vi "Actor Core.vi"(8 "error in":errorcluster, 11 "RandomDataChart in":refnum<class "AutoRegPanel.lvclass">) -> (0 "error out":errorcluster, 3 "Actor out":refnum<class "Actor.lvclass">)   [LabVIEW 2015, in "TestActors.lvlib" / "AutoRegPanel.lvclass"]
doc: "(<B>Filename</B>: Actor Framework.lvlib:Actor.lvclass:Actor Core.vi)\n\nReceives messages to the actor, reacts to them, and initiates any error handling that may shut the actor down.\n\nDescendant classes may override this VI to append parallel tasks for the actor to complete while it handles messages. Overrides use the Call Parent Method node."
uses:
  AutoRegPanel.lvclass
  <vilib>/ActorFramework/Actor/Actor.lvclass
  <vilib>/ActorFramework/Actor/Actor.lvclass/Actor.ctl
  <vilib>/ActorFramework/Message Enqueuer/Message Enqueuer.lvclass/Message Enqueuer.ctl
  <vilib>/ActorFramework/Message Enqueuer/Init from Existing Queue.vi
  IViewable/IViewable/IViewable.lvclass
  <vilib>/ActorFramework/Message Enqueuer/Message Enqueuer.lvclass
  AutoRegistration/AutoRegistration/AutoRegistration.lvclass
  AutoRegistration/ActorAutoRegistration Messages/BooleanValueMsg/BooleanValueMsg.lvclass
panel:
  in  "Whitaker":bool caption="Latch When Released"
  in  "Walton":bool caption="Latch Until Released"
  in  "Launch Dialog":bool
  in  "Guthrie":bool caption="Switch Until Released"
  in  "Harrelson":bool caption="Switch When Released"
  in  "Gump":bool caption="Latch When Pressed"
  in  "Wilson":bool caption="Switch When Pressed"
  # "An actor implementing\ngeneral auto-reg in core"
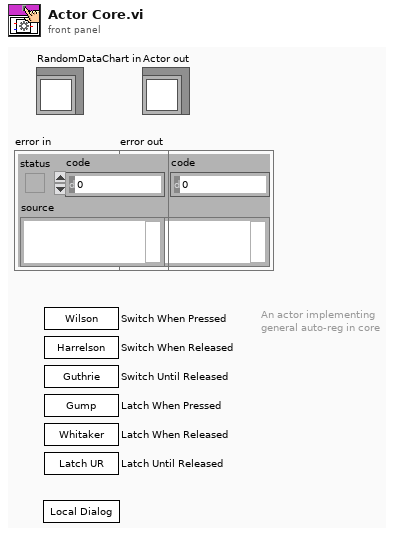
[diagram p1: front panel]
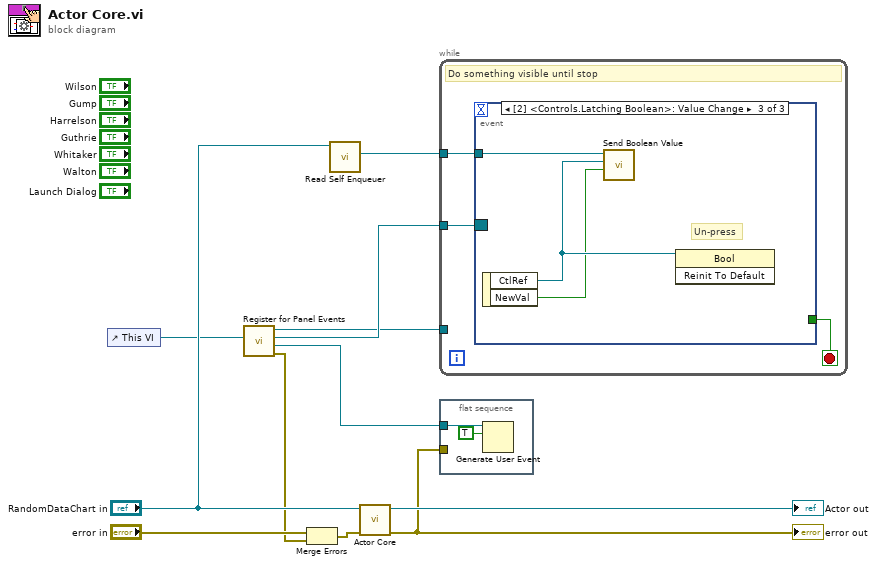
[diagram p0: block diagram]
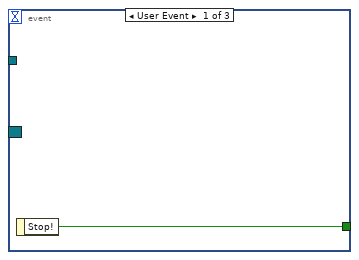
[diagram p2: hidden frame]
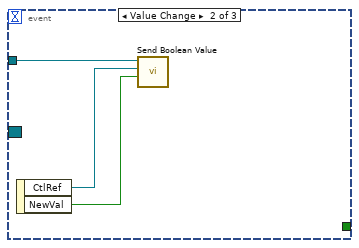
[diagram p3: hidden frame]
diagram:
  n1 = control-ref of="This VI"() -> (w6:refnum<vi>)
  n2 = call "Register for Panel Events.vi"("VI Refnum (Caller)"=w6) -> ("error out"=w3:errorcluster, "Stop! Event"=w5:refnum<user-event>, "Event Registration Refnum"=w2:refnum<event-registration>, "AbstractAutoRegistration out"=w1:refnum<class "AutoRegistration.lvclass">)  [unwired: 7 in]
  n3 = Merge Errors("error in", w3) -> (w4:errorcluster)
  n4 = call <vilib>:"Read Self Enqueuer.vi"("Actor"="RandomDataChart in") -> ("Self Enqueuer"=w7:refnum<class "Message Enqueuer.lvclass">)  [unwired: 10 in]
  n5 = call-parent "Actor Core.vi"("error in"=w4, "IViewable In"="RandomDataChart in") -> ("error out"=w9:errorcluster, "Actor out"=→"Actor out":refnum<class "Actor.lvclass">)  [unwired: 8 in]
  "error out" <- w9
  n6 = while {
    tunnel: w2 -> [w14]
    tunnel: w7 -> [w12]
    tunnel: w1 -> [_]
    stop <- w13 stop-if-true
    # "Do something visible until stop"
    n7 = event shown="[2] <Controls.Latching Boolean>: Value Change" {
      selector: w14 -> [_ _ _]
      dyn-events: _ -> [_ _ _]
      timeout: _ -> [_ _ _]
      tunnel: [w15 _ _] -> w13
      tunnel: w12 -> [_ w18 w21]
      event User Event {
        n8 = event-data() -> ("Stop!"=w15:bool)  [unwired: 1 in]
      }
      event Value Change {
        n9 = event-data() -> ("CtlRef"=w17:refnum<vi>, "NewVal"=w16:bool)  [unwired: 1 in]
        n10 = call "Send Boolean Value.vi"("Value"=w16, "Boolean Refnum"=w17, "Message Enqueuer in"=w18) -> ()  [unwired: 8 in, 1 out]
      }
      event Value Change {
        # "Un-press"
        n11 = event-data() -> ("CtlRef"=w20:refnum<vi>, "NewVal"=w19:bool)  [unwired: 1 in]
        n12 = call "Send Boolean Value.vi"("Value"=w19, "Boolean Refnum"=w20, "Message Enqueuer in"=w21) -> ()  [unwired: 8 in, 1 out]
        n13 = invoke class="Bool" method="Reinit To Default"(reference=w20) -> ()  [unwired: 2 in, 3 out]
      }
    }
  }
  n14 = flat-sequence {
    tunnel: w5 -> [w23]
    tunnel: w9 -> [_]
    frame #0 {
      n15 = Generate User Event(user event=w23, event data cluster=TRUE ("event data")) -> ()  [unwired: 2 in, 2 out]
    }
  }
